vi "Configuration 1.3 Finalize.vi"(8 "error in (no error)":errorcluster, 10 "file version (x.y)":T2, 11 "configuration 1.3":T1) -> (0 "error out":errorcluster, 2 "final file version":T2, 3 "configuration json":string)   [LabVIEW 2020, in "DSF Core.lvlib" / "Configuration Session.lvclass"]
uses:
  Configuration Session.lvclass
  Typedefs/DSF Version Info.ctl
  DSF Core.lvlib
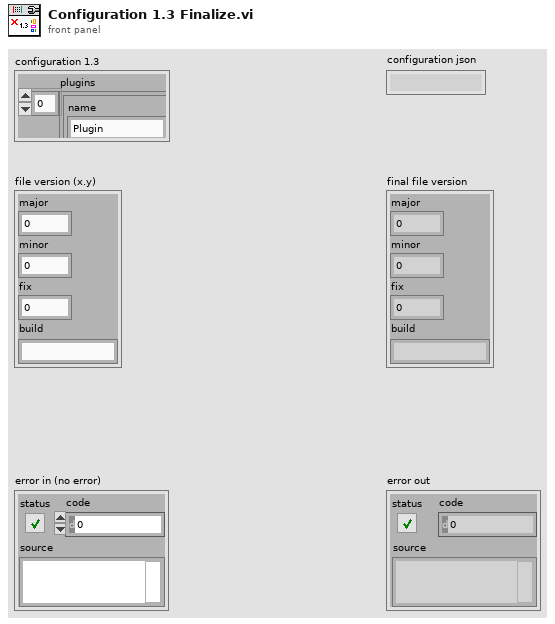
[diagram p1: front panel]
types:
  T1 = cluster{"plugins":cluster{"name":string, "components":string[], "cycle timing":cluster{"priority":u64, "decimation":u64, "offset":u64}, "threads":cluster{"processor":i32, "priority offset":i16, "settings":cluster{"component":string, "name":string, "values":cluster{"key":string, "value":string}[]}[]}[], "transfer groups":cluster{"name":string, "direction":enum8{"Tx", "Rx"}, "cycle timing":cluster{"priority":u64, "decimation":u64, "offset":u64}, "thread index":u8, "settings":cluster{"component":string, "name":string, "values":cluster{"key":string, "value":string}[]}[], "transfers":cluster{"name":string, "byte order":enum8{"big-endian", "little-endian"}, "settings":cluster{"component":string, "name":string, "values":cluster{"key":string, "value":string}[]}[], "channels":cluster{"string offset":u64, "name":string, "units":string, "engine data type":enum8{"Bool", "SGL", "DBL", "I8", "I16", "I32", "I64", "U8", "U16", "U32", "U64"}, "string data type":enum8{"Bool", "SGL", "DBL", "I8", "I16", "I32", "I64", "U8", "U16", "U32", "U64"}, "settings":cluster{"component":string, "name":string, "values":cluster{"key":string, "value":string}[]}[]}[]}[], "timeout behavior":enum8{"Increment Late Count", "Throw Error"}, "enable buffer conversion":bool}[], "settings":cluster{"component":string, "name":string, "values":cluster{"key":string, "value":string}[]}[]}[]}
  T2 = typedef "DSF Core.lvlib/DSF Version Info.ctl" = cluster{"major":u32, "minor":u32, "fix":u32, "build":string}
  T3 = cluster{"plugins":cluster{"name":string, "components":string[], "cycle timing":cluster{"priority":u64, "decimation":u64, "offset":u64}, "threads":cluster{"processor":i32, "priority offset":i16, "settings":cluster{"component":string, "name":string, "values":cluster{"key":string, "value":string}[]}[]}[], "transfer groups":cluster{"name":string, "direction":enum8{"Tx", "Rx"}, "cycle timing":cluster{"priority":u64, "decimation":u64, "offset":u64}, "thread index":i32, "settings":cluster{"component":string, "name":string, "values":cluster{"key":string, "value":string}[]}[], "transfers":cluster{"name":string, "byte order":enum8{"big-endian", "little-endian"}, "settings":cluster{"component":string, "name":string, "values":cluster{"key":string, "value":string}[]}[], "channels":cluster{"string offset":u64, "name":string, "units":string, "engine data type":enum8{"Bool", "SGL", "DBL", "I8", "I16", "I32", "I64", "U8", "U16", "U32", "U64"}, "string data type":enum8{"Bool", "SGL", "DBL", "I8", "I16", "I32", "I64", "U8", "U16", "U32", "U64"}, "settings":cluster{"component":string, "name":string, "values":cluster{"key":string, "value":string}[]}[]}[]}[], "timeout behavior":enum8{"Increment Late Count", "Throw Error"}}[], "settings":cluster{"component":string, "name":string, "values":cluster{"key":string, "value":string}[]}[]}[]}
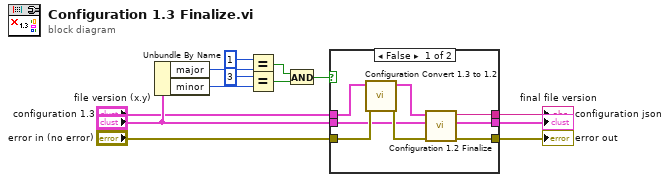
[diagram p0: block diagram]
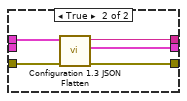
[diagram p2: hidden frame]
diagram:
  n1 = Unbundle By Name("file version (x.y)") -> ("major"=w12:u32, "minor"=w13:u32)
  n2 = Equal?(x=u32 1, y=w12) -> (x = y?=w8:bool)
  n3 = Equal?(x=u32 3, y=w13) -> (x = y?=w9:bool)
  n4 = And(x=w8, y=w9) -> (x .and. y?=w7:bool)
  n5 = case shown="False" w7 {
    tunnel: "error in (no error)" -> [w18 w26]
    tunnel: "configuration 1.3" -> [w14 w25]
    tunnel: [w21 w24] -> w4
    tunnel: "file version (x.y)" -> [w15 _]
    tunnel: [w20 w23] -> w5
    tunnel: [w19 w22] -> w2
    frame False {
      n6 = call "Configuration Convert 1.3 to 1.2.vi"("error in (no error)"=w18, "configuration 1.3"=w14) -> ("error out"=w16:errorcluster, "configuration 1.2"=w17:T3)  [unwired: 8 in]
      n7 = call "Configuration 1.2 Finalize.vi"("error in (no error)"=w16, "file version (x.y)"=w15, "configuration 1.2"=w17) -> ("error out"=w21:errorcluster, "final file version"=w19:T2, "configuration json"=w20:string)  [unwired: 6 in]
    }
    frame True {
      n8 = call "Configuration 1.3 JSON Flatten.vi"("error in (no error)"=w26, "configuration 1.3"=w25) -> ("error out"=w24:errorcluster, "dsf version"=w22:T2, "configuration json"=w23:string)  [unwired: 7 in]
    }
  }
  "error out" <- w4
  "final file version" <- w2
  "configuration json" <- w5
